vi "API_Edit_Window.vi"(1 "VI Path":path) -> (0 "VI Reference":refnum<vi>)   [LabVIEW 2011]
doc: "This VI initializes the calling API VI's front panel window."
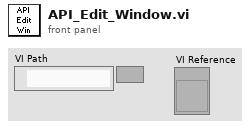
[diagram p1: front panel]
types:
  T1 = enum32{"Invalid", "Default", "Floating", "Floating/Auto-Hide", "Modal"}
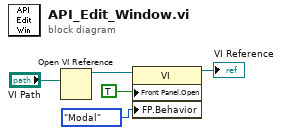
[diagram p0: block diagram]
diagram:
  n1 = Open VI Reference(vi path="VI Path") -> (vi reference=w3:refnum<vi>)  [unwired: 1 in, 5 out]
  n2 = property class="VI"(reference=w3, "Front Panel.Open"=TRUE ("Front Panel Window:Open"), "FP.Behavior"=T1."Modal" ("Front Panel Window:Behavior")) -> (reference out=→"VI Reference":refnum<vi>)  [unwired: 1 in, 1 out]
